vi "p2pgenerator.vi"(6 "whole time for p2p":i32, 8 "ts":dbl, 9 "p_end":dbl, 10 "a_max":dbl, 11 "v_max":dbl) -> (0 "jerk":dbl[](array[numeric]), 1 "a":dbl[](array[numeric]), 2 "v":dbl[](array[numeric]), 3 "s":dbl[](array[numeric]))   [LabVIEW 2020]
uses:
  <vilib>/imath/engines/lvmath2/RunTimeEngine/BuiltInFunctions/mod/NIMS_mod_no_size_check.vi
  <instcachedir>/0/NIMS_mod_no_size_check_5393E3382FD241D281EEB71DA286C65B.lvgen/NIMS_mod_no_size_check_5393E3382FD241D281EEB71DA286C65B_001.vi
  <vilib>/imath/engines/lvmath2/RunTimeEngine/IndexReplace/NIMS V(S)=S.vi
  <instcachedir>/0/NIMS V(S)=S_36728E0438CF49488BD4AB9ABCA5ECA4.lvgen/NIMS V(S)=S_36728E0438CF49488BD4AB9ABCA5ECA4_000.vi
  <vilib>/imathl/engines/lvmath/Functions/Error Handling/Create Error.vi
  <vilib>/imath/engines/lvmath2/RunTimeEngine/NodeEndStatement/NIMS_NodeEndStatement_Output.vi
  <instcachedir>/0/NIMS_NodeEndStatement_Output_53EC0D466D134D7ABD903AC30B43404B.lvgen/NIMS_NodeEndStatement_Output_53EC0D466D134D7ABD903AC30B43404B_005.vi
  <vilib>/imath/engines/lvmath2/RunTimeEngine/ErrorHandling/NIMS_Finalize Error.vi
  <vilib>/imath/engines/lvmath2/RunTimeEngine/VariableToken/NIMS_VariableToken_CondDefinedDefinedByReplace.vi
  <instcachedir>/0/NIMS_VariableToken_CondDefinedDefinedByReplace_D162CFFC24174562A9FEA619A91E1A56.lvgen/NIMS_VariableToken_CondDefinedDefinedByReplace_D162CFFC24174562A9FEA619A91E1A56_003.vi
  <vilib>/imath/engines/lvmath2/RunTimeEngine/VariableToken/NIMS_VariableToken_CondDefined.vi
  <instcachedir>/0/NIMS_VariableToken_CondDefined_537E119D71C74F9D9452D6FF923F1E1F.lvgen/NIMS_VariableToken_CondDefined_537E119D71C74F9D9452D6FF923F1E1F_004.vi
panel:
  out "Waveform Chart":dbl[](graph)
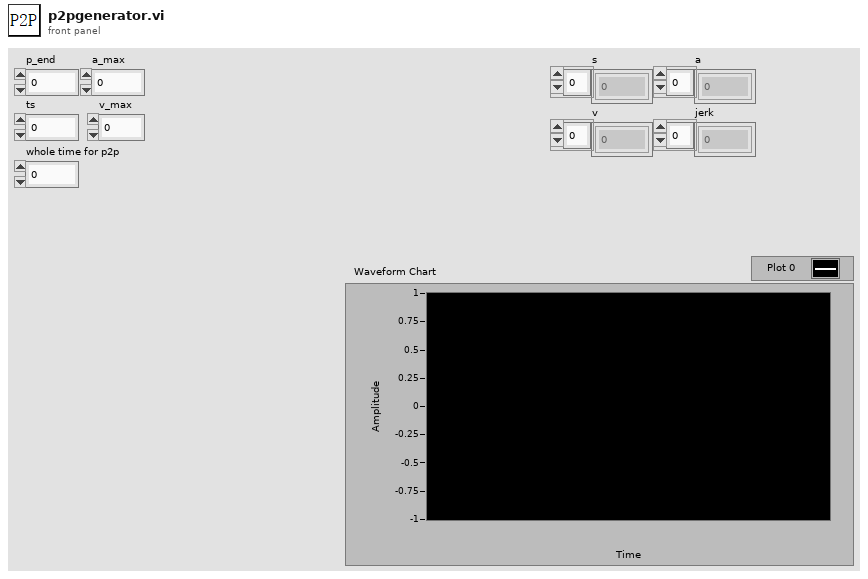
[diagram p1: front panel]
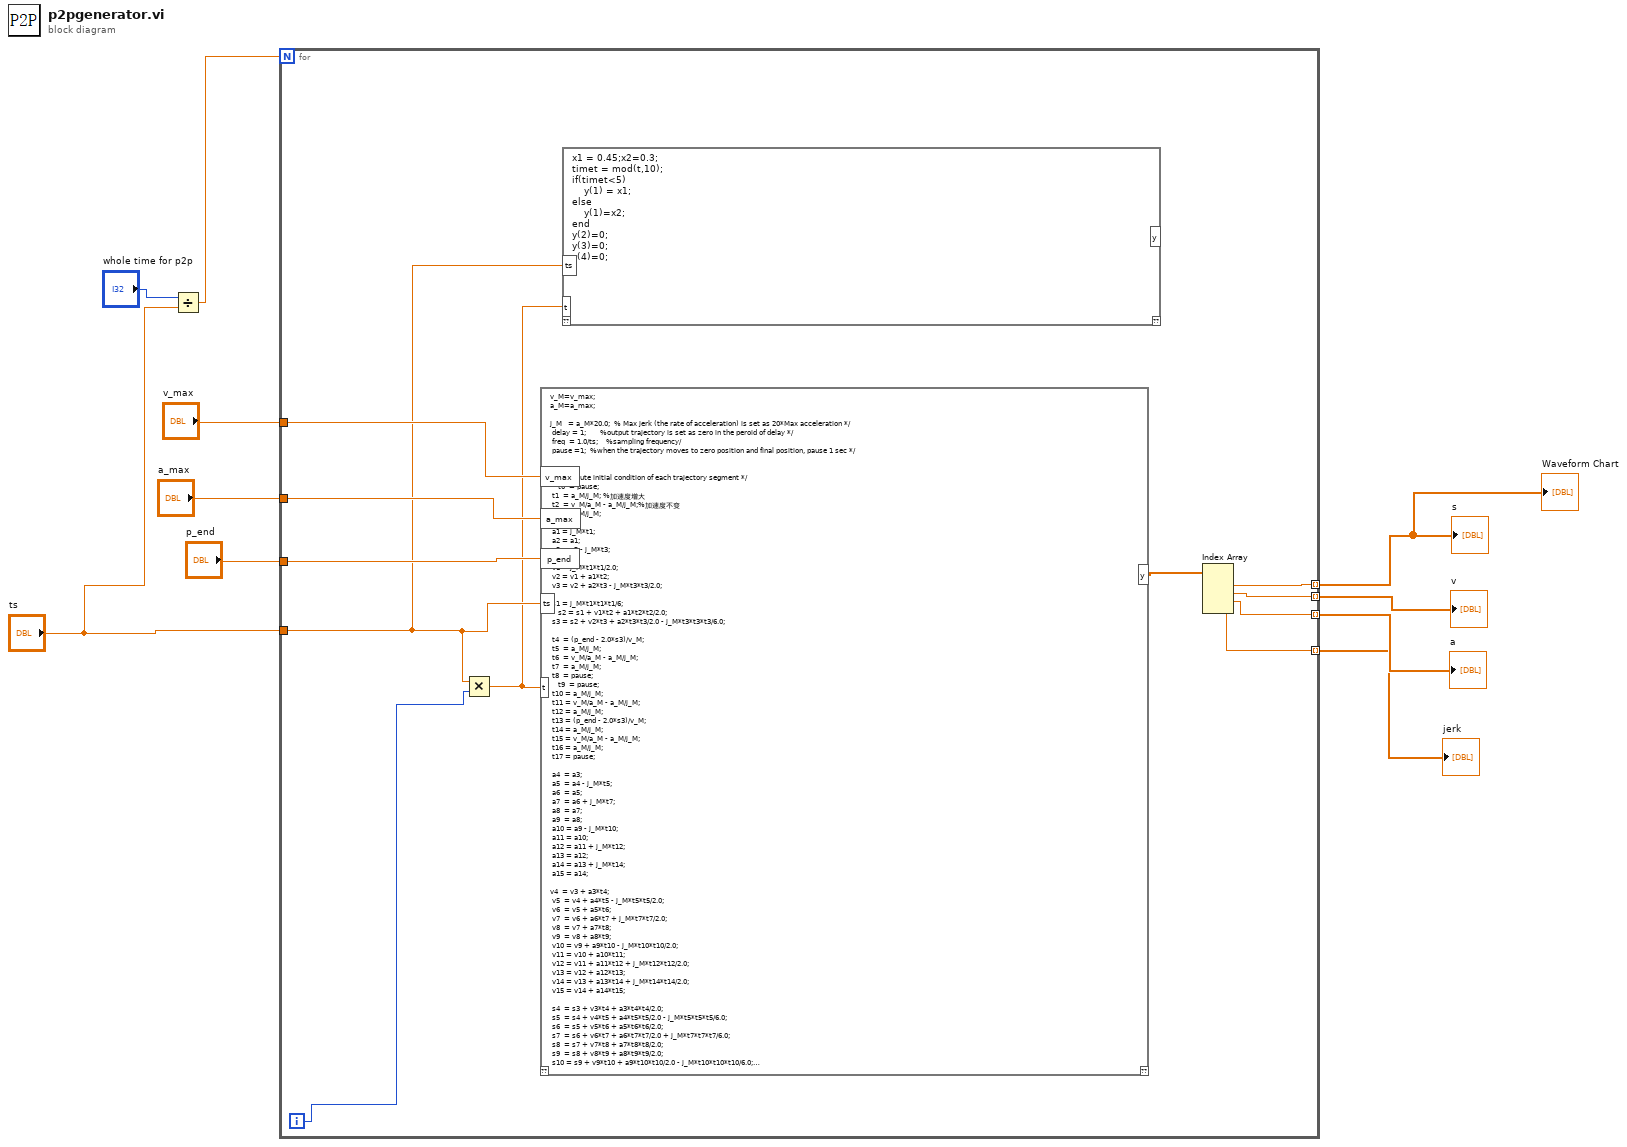
[diagram p0: block diagram]
diagram:
  n1 = Divide(x="whole time for p2p", y="ts") -> (x/y=w2:dbl)
  n2 = for {
    N: w2 -> [_]
    tunnel: [w21] -> w1 mode=indexing
    tunnel: [w20] -> w7 mode=indexing
    tunnel: [w19] -> w6 mode=indexing
    tunnel: [w18] -> w5 mode=indexing
    tunnel: "v_max" -> [w16]
    tunnel: "a_max" -> [w15]
    tunnel: "p_end" -> [w14]
    tunnel: "ts" -> [w13]
    i -> [w17]
    n3 = Multiply(x=w13, y=w17) -> (x*y=w12:dbl)
    n4 = mathscript code="v_M=v_max;\na_M=a_max;\n\nj_M\t  = a_M*20.0;  % Max jerk (the rate of acceleration) is set as 20*Max acceleration */\n\tdelay = 1;       %output trajectory is set as zero in the peroid of delay */\n\tfreq  = 1.0/ts;    %sampling frequency/\n\tpause =1;\t\t%when the trajectory moves to zero position and final position, pause 1 sec */\n\n\n\t% compute initial condition of each trajectory segment */\n    t0  = pause;\n\tt1  = a_M/j_M; %加速度增大\n\tt2  = v_M/a_M - a_M/j_M;%加速度不变\n\tt3  = a_M/j_M;\n\n\ta1 = j_M*t1;\n\ta2 = a1;\n\ta3 = a2 - j_M*t3;\n\n\tv1 = j_M*t1*t1/2.0;\n\tv2 = v1 + a1*t2;\n\tv3 = v2 + a2*t3 - j_M*t3*t3/2.0;\n\n s1 = j_M*t1*t1*t1/6;\n    s2 = s1 + v1*t2 + a1*t2*t2/2.0;\n\ts3 = s2 + v2*t3 + a2*t3*t3/2.0 - j_M*t3*t3*t3/6.0;\n\n\tt4  = (p_end - 2.0*s3)/v_M;\n\tt5  = a_M/j_M;\n\tt6  = v_M/a_M - a_M/j_M;\n\tt7  = a_M/j_M;\n\tt8  = pause;\n    t9  = pause;\n\tt10 = a_M/j_M;\n\tt11 = v_M/a_M - a_M/j_M;\n\tt12 = a_M/j_M;\n\tt13 = (p_end - 2.0*s3)/v_M;\n\tt14 = a_M/j_M;\n\tt15 = v_M/a_M - a_M/j_M;\n\tt16 = a_M/j_M;\n\tt17 = pause;\n\n\ta4  = a3;\n\ta5  = a4 - j_M*t5;\n\ta6  = a5;\n\ta7  = a6 + j_M*t7;\n\ta8  = a7;\n\ta9  = a8;\n\ta10 = a9 - j_M*t10;\n\ta11 = a10;\n\ta12 = a11 + j_M*t12;\n\ta13 = a12;\n\ta14 = a13 + j_M*t14;\n\ta15 = a14;\n\nv4  = v3 + a3*t4;\n\tv5  = v4 + a4*t5 - j_M*t5*t5/2.0;\n\tv6  = v5 + a5*t6;\n\tv7  = v6 + a6*t7 + j_M*t7*t7/2.0;\n\tv8  = v7 + a7*t8;\n\tv9  = v8 + a8*t9;\n\tv10 = v9 + a9*t10 - j_M*t10*t10/2.0;\n\tv11 = v10 + a10*t11;\n\tv12 = v11 + a11*t12 + j_M*t12*t12/2.0;\n\tv13 = v12 + a12*t13;\n\tv14 = v13 + a13*t14 + j_M*t14*t14/2.0;\n\tv15 = v14 + a14*t15;\n\n\ts4  = s3 + v3*t4 + a3*t4*t4/2.0;\n\ts5  = s4 + v4*t5 + a4*t5*t5/2.0 - j_M*t5*t5*t5/6.0;\n\ts6  = s5 + v5*t6 + a5*t6*t6/2.0;\n\ts7  = s6 + v6*t7 + a6*t7*t7/2.0 + j_M*t7*t7*t7/6.0;\n\ts8  = s7 + v7*t8 + a7*t8*t8/2.0;\n\ts9  = s8 + v8*t9 + a8*t9*t9/2.0;\n\ts10 = s9 + v9*t10 + a9*t10*t10/2.0 - j_M*t10*t10*t10/6.0;\n\ts11 = s10 + v10*t11 + a10*t11*t11/2.0;\n\ts12 = s11 + v11*t12 + a11*t12*t12/2.0 + j_M*t12*t12*t12/6.0;\n\ts13 = s12 + v12*t13 + a12*t13*t13/2.0;\n\ts14 = s13 + v13*t14 + a13*t14*t14/2.0 + j_M*t14*t14*t14/6.0;\n\ts15 = s14 + v14*t15 + a14*t15*t15/2.0;\n\ts16 = s15 + v15*t16 + a15*t16*t16/2.0 - j_M*t16*t16*t16/6.0;\n\n\tT0  = t0;\n\tT1  = T0 + t1;\n\tT2  = T1 + t2;\n\tT3  = T2 + t3;\n\tT4  = T3 + t4;\n\tT5  = T4 + t5;\n\tT6  = T5 + t6;\n\tT7  = T6 + t7;\n\tT8  = T7 + t8;\n\tT9  = T8 + t9;\n\tT10 = T9 + t10;\n\tT11 = T10 + t11;\n\tT12 = T11 + t12;\n\tT13 = T12 + t13;\n\tT14 = T13 + t14;\n\tT15 = T14 + t15;\n\tT16 = T15 + t16;\n\tT17 = T16 + t17;\n\n%/* generate trajectory */\n  if(t<=delay)\n\ty(4) = 0.0;\t   % /* jerk */\n\ty(2) = 0.0;\t\t%/* acceleration */\n    y(3) = 0.0;\t\t%/* velocity */\n\ty(1) = 0.0;\t\t%/* position */\n  else\n% \t q0\t  = *uPtrs[0];%q0 is what?\n\t T\t  = T17*freq;\n     tt   = (t-delay)*freq;\n     rt   = mod(tt,T);\n     rrt  = rt/freq;\n  \n    if(rt<=T0*freq)\n\t\ty(4) = 0.0;\t   % /* jerk */\n\ty(3) = 0.0;\t\t%/* acceleration */\n    y(2) = 0.0;\t\t%/* velocity */\n\ty(1) = 0.0;\t\t%/* position */\n    end\n\n    if(rt>T0*freq & rt<=T1*freq)\n\t\ty(4) = j_M;\n\t\t y(3) = j_M*(rrt-T0);\n\t\t y(2) = j_M*(rrt-T0)*(rrt-T0)/2.0;\n\t\t y(1) = j_M*(rrt-T0)*(rrt-T0)*(rrt-T0)/6.0;\n    end\n\t\t\n\n\tif(rt>T1*freq & rt<=T2*freq)\n\t\ty(4) = 0.0;\n\t\t y(3) = a1;\n\t\t y(2) = v1 + a1*(rrt-T1);\n\t\t y(1) = s1 + v1*(rrt-T1) + a1*(rrt-T1)*(rrt-T1)/2.0;\n    end\n\t\t\n\n\tif(rt>T2*freq & rt<=T3*freq)\n\t\ty(4) = -j_M;\n\t\t y(3) = a2 - j_M*(rrt-T2);\n\t\t y(2) = v2 + a2*(rrt-T2) - j_M*(rrt-T2)*(rrt-T2)/2.0;\n\t\t y(1) = s2 + v2*(rrt-T2) + a2*(rrt-T2)*(rrt-T2)/2.0 - j_M*(rrt-T2)*(rrt-T2)*(rrt-T2)/6.0;\n    end\n\t\t\n\n\tif(rt>T3*freq & rt<=T4*freq)\n\t\ty(4) = 0.0;\n\t\t y(3) = a3;\n\t\t y(2) = v3 + a3*(rrt-T3);\n\t\t y(1) = s3 + v3*(rrt-T3) + a3*(rrt-T3)*(rrt-T3)/2.0;\n    end\n\t\t\n\n\tif(rt>T4*freq & rt<=T5*freq)\n\t\ty(4) = -j_M;\n\t\t y(3) = a4 - j_M*(rrt-T4);\n\t\t y(2) = v4 + a4*(rrt-T4) - j_M*(rrt-T4)*(rrt-T4)/2.0;\n\t\t y(1) = s4 + v4*(rrt-T4) + a4*(rrt-T4)*(rrt-T4)/2.0 - j_M*(rrt-T4)*(rrt-T4)*(rrt-T4)/6.0;\n    end\n\t\t\n\n    if(rt>T5*freq & rt<=T6*freq)\n\t\ty(4) = 0;\n\t\t y(3) = a5;\n\t\t y(2) = v5 + a5*(rrt-T5);\n\t\t y(1) = s5 + v5*(rrt-T5) + a5*(rrt-T5)*(rrt-T5)/2.0;\n    end\n\t\t\n\n    if(rt>T6*freq & rt<=T7*freq)\n\t\ty(4) = j_M;\n\t\t y(3) = a6 + j_M*(rrt-T6);\n\t\t y(2) = v6 + a6*(rrt-T6) + j_M*(rrt-T6)*(rrt-T6)/2.0;\n\t\t y(1) = s6 + v6*(rrt-T6) + a6*(rrt-T6)*(rrt-T6)/2.0 + j_M*(rrt-T6)*(rrt-T6)*(rrt-T6)/6.0;\n    end\n\t\t\n\n\tif(rt>T7*freq & rt<=T8*freq)\n\t\ty(4) = 0.0;\n\t\t y(3) = 0.0;\n\t\t y(2) = 0.0;\n\t\t y(1) = s7;\n    end\n\t\t\n\n\tif(rt>T8*freq & rt<=T9*freq)\n\t\ty(4) = 0.0;\n\t\t y(3) = 0.0;\n\t\t y(2) = 0.0;\n\t\t y(1) = s8;\n    end\n\t\t\n\n\tif(rt>T9*freq & rt<=T10*freq)\n\t\ty(4) = -j_M;\n\t\t y(3) = a9 - j_M*(rrt-T9);\n\t\t y(2) = v9 + a9*(rrt-T9) - j_M*(rrt-T9)*(rrt-T9)/2.0;\n\t\t y(1) = s9 + v9*(rrt-T9) + a9*(rrt-T9)*(rrt-T9)/2.0 - j_M*(rrt-T9)*(rrt-T9)*(rrt-T9)/6.0;\n    end\n\t\t\n\n\tif(rt>T10*freq & rt<=T11*freq)\n\t\ty(4) = 0.0;\n\t\t y(3) = a10;\n\t\t y(2) = v10 + a10*(rrt-T10);\n\t\t y(1) = s10 + v10*(rrt-T10) + a10*(rrt-T10)*(rrt-T10)/2.0;\n    end\n\t\t\n\n\n   if(rt>T11*freq & rt<=T12*freq)\n\t\ty(4) = j_M;\n\t\t y(3) = a11 + j_M*(rrt-T11);\n\t\t y(2) = v11 + a11*(rrt-T11) + j_M*(rrt-T11)*(rrt-T11)/2.0;\n\t\t y(1) = s11 + v11*(rrt-T11) + a11*(rrt-T11)*(rrt-T11)/2.0 + j_M*(rrt-T11)*(rrt-T11)*(rrt-T11)/6.0;\n   end\n\t\t\n  \n   if(rt>T12*freq & rt<=T13*freq)\n\t\ty(4) = 0;\n\t\t y(3) = a12;\n\t\t y(2) = v12 + a12*(rrt-T12);\n\t\t y(1) = s12 + v12*(rrt-T12) + a12*(rrt-T12)*(rrt-T12)/2.0;\n   end\n\t\t\n\n   if(rt>T13*freq & rt<=T14*freq)\n\t\ty(4) = j_M;\n\t\t y(3) = a13 + j_M*(rrt-T13);\n\t\t y(2) = v13 + a13*(rrt-T13) + j_M*(rrt-T13)*(rrt-T13)/2.0;\n\t\t y(1) = s13 + v13*(rrt-T13) + a13*(rrt-T13)*(rrt-T13)/2.0 + j_M*(rrt-T13)*(rrt-T13)*(rrt-T13)/6.0;\n   end\n\t\t\n\n   if(rt>T14*freq & rt<=T15*freq)\n\t\ty(4) = 0.0;\n\t\t y(3) = a14;\n\t\t y(2) = v14 + a14*(rrt-T14);\n\t\t y(1) = s14 + v14*(rrt-T14) + a14*(rrt-T14)*(rrt-T14)/2.0;\n   end\n\t\t\n\n   if(rt>T15*freq & rt<=T16*freq)\n\t\ty(4) = -j_M;\n\t\t y(3) = a15 - j_M*(rrt-T15);\n\t\t y(2) = v15 + a15*(rrt-T15) - j_M*(rrt-T15)*(rrt-T15)/2.0;\n\t\t y(1) = s15 + v15*(rrt-T15) + a15*(rrt-T15)*(rrt-T15)/2.0 - j_M*(rrt-T15)*(rrt-T15)*(rrt-T15)/6.0;\n   end\n\t\t\n\n   if(rt>T16*freq & rt<=T17*freq)\n\t\ty(4) = 0.0;\n\t\t y(3) = 0.0;\n\t\t y(2) = 0.0;\n\t\t y(1) = s16;\n   end  \n  end"("v_max"=w16, "a_max"=w15, "p_end"=w14, "ts"=w13, "t"=w12) -> ("y"=w11:dbl[])  [unwired: 1 in, 1 out]
    n5 = mathscript code="x1 = 0.45;x2=0.3;\ntimet = mod(t,10);\nif(timet<5)\n    y(1) = x1;\nelse\n    y(1)=x2;\nend\ny(2)=0;\ny(3)=0;\ny(4)=0;"("ts"=w13, "t"=w12) -> ()  [unwired: 1 in, 2 out]
    n6 = Index Array(array=w11) -> (element #1=w21:dbl, element #2=w20:dbl, element #3=w19:dbl, element #4=w18:dbl)  [unwired: 4 in]
  }
  "s" <- w1
  "v" <- w7
  "a" <- w6
  "jerk" <- w5
  "Waveform Chart" <- w1
